vi "Handle Response.vi"(7 "Inputs":T2, 8 "error in (no error)":errorcluster, 11 "FileExistChecker in":refnum<class "FileExistChecker.lvclass">) -> (0 "error out":errorcluster, 5 "Outputs":T1)   [LabVIEW 2020, in "HTTP Server.lvlib" / "FileExistChecker.lvclass"]
uses:
  FileExistChecker.lvclass
  Response Inputs.ctl
  Values/Values.lvclass
  <vilib>/IlluminatedG/IG HTTP Utils/HTTP Utils/Request/Request.lvclass
  <vilib>/IlluminatedG/IG HTTP Utils/HTTP Utils/Response/Response.lvclass
  Session/Session.lvclass
  Response Outputs.ctl
  File Response/File Response.lvclass
  FileExistChecker.lvclass/FileExistChecker.ctl
  HTTP Server.lvlib
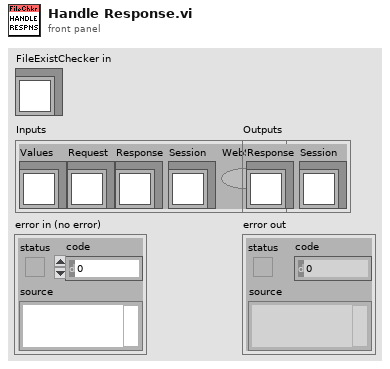
[diagram p1: front panel]
types:
  T1 = typedef "HTTP Server.lvlib/Response Outputs.ctl" = cluster{"Response":refnum<class "Response.lvclass">, "Session":refnum<class "Session.lvclass">}
  T2 = typedef "HTTP Server.lvlib/Response Inputs.ctl" = cluster{"Values":refnum<class "Values.lvclass">, "Request":refnum<class "Request.lvclass">, "Response":refnum<class "Response.lvclass">, "Session":refnum<class "Session.lvclass">, "WebSocket":bool}
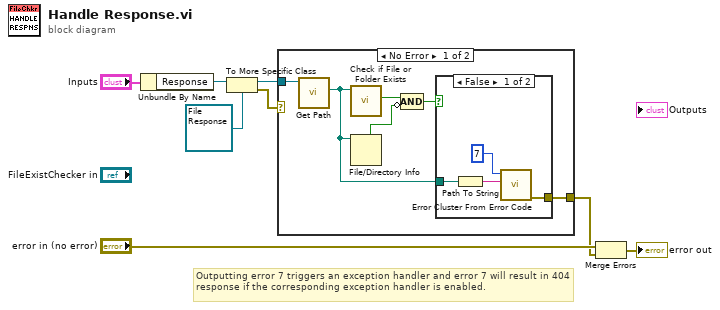
[diagram p0: block diagram]
diagram:
  # "Outputting error 7 triggers an exception handler and error 7 will result in 404 response if the corresponding exception handler is enabled."
  n1 = Unbundle By Name("Inputs") -> ("Response"=w1:refnum<class "Response.lvclass">)
  n2 = To More Specific Class(target class=refnum<class "File Response.lvclass"> refnum ("HTTP Server.lvlib:File Response.lvclass"), reference=w1) -> (specific class reference=w5:refnum<class "File Response.lvclass">, error out=w6:errorcluster)  [unwired: 1 in]
  n3 = case shown="No Error" w6 {
    tunnel: w5 -> [w14 _]
    tunnel: [w12 _] -> w3
    frame No Error {
      n4 = call "Get Path.vi"("File Response in"=w14) -> ("Path"=w11:path)  [unwired: 8 in, 2 out]
      n5 = call <vilib>:"Check if File or Folder Exists.vi"("path"=w11) -> ("file or folder exists?"=w13:bool)  [unwired: 8 in, 2 out]
      n6 = File/Directory Info(path=w11) -> (directory=w9:bool)  [unwired: 1 in, 6 out]
      n7 = Compound Arithmetic op=AND(w13, invert w9) -> (w10:bool)
      n8 = case shown="False" w10 {
        tunnel: w11 -> [w17 _]
        tunnel: [w15 _] -> w12
        frame False {
          n9 = Path To String(path=w17) -> (string=w16:string)
          n10 = call <vilib>:"Error Cluster From Error Code.vi"("error message (\"\")"=w16, "error code (0)"=7) -> ("error out"=w15:errorcluster)  [unwired: 7 in]
        }
        frame True {
        }
      }
    }
    frame Error {
    }
  }
  n11 = Merge Errors("error in (no error)", w3) -> (→"error out":errorcluster)
